vi "GetSensorGroupEndpoints.vi"(11 "SensorGroupId":string) -> (3 "Endpoints out":T1[](array[typedef]))   [LabVIEW 2017, in "DeviceModelHelpers.lvlib"]
uses:
  <vilib>/addons/InsightCM/Utilities/DeviceModelHelpers/DeviceModelHelpers.lvlib
  <vilib>/addons/InsightCM/MessageBus/Base/controls/WirelessEndpoint.ctl
  <vilib>/addons/InsightCM/MessageBus/Base/controls/KeyValuePair.ctl
  <vilib>/addons/InsightCM/MessageBus/Base/controls/WirelessChannel.ctl
  <vilib>/addons/InsightCM/Utilities/GlobalConfiguration/GlobalConfiguration.lvlib
  <vilib>/addons/InsightCM/Utilities/PropertyHelpers/PropertyHelpers.lvlib
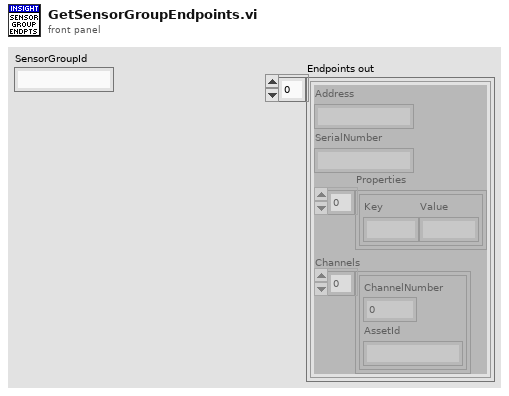
[diagram p1: front panel]
types:
  T1 = typedef "WirelessEndpoint.ctl" = cluster{"Address":string, "SerialNumber":string, "Properties":T2[], "Channels":T3[]}
  T2 = typedef "KeyValuePair.ctl" = cluster{"Key":string, "Value":string}
  T3 = typedef "WirelessChannel.ctl" = cluster{"ChannelNumber":i32, "AssetId":string}
  T4 = typedef "R2_Device.ctl" = cluster{"Id":string, "Name":string, "DeviceType":string, "HardwareName":string, "IpAddress":string, "HardwareInfo":T2[], "ApplicationType":string, "ApplicationVersion":string, "EquipmentIds":string[], "ConfigurationVersion":string, "State":T5, "Properties":T2[], "DataGroups":T6[], "BurstModeTrigger":T10, "SensorGroups":T11[], "Endpoints":T1[]}
  T5 = typedef "DeviceState.ctl" = cluster{"Disabled":bool}
  T6 = typedef "R2_DataGroup.ctl" = cluster{"Name":string, "OperatingStates":T7[], "Properties":T2[], "EquipmentIds":string[], "AssetNodeId":string}
  T7 = typedef "OperatingState.ctl" = cluster{"Name":string, "Properties":T2[], "Triggers":T8[]}
  T8 = typedef "Trigger.ctl" = cluster{"Type":string, "Expression":string, "Conditions":T9[]}
  T9 = typedef "Condition.ctl" = cluster{"Source":string, "Type":string, "Operator":string, "CompareTo":string, "DwellSeconds":dbl}
  T10 = typedef "BurstModeTrigger.ctl" = cluster{"Trigger":T8, "SampleRate":string, "AcquisitionLength":string}
  T11 = typedef "DeviceSensorGroup.ctl" = cluster{"EquipId":string, "SensorGroupId":string}
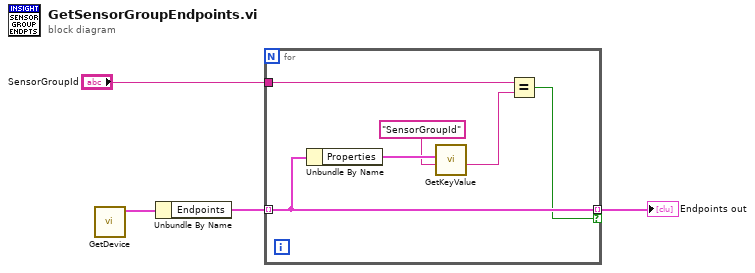
[diagram p0: block diagram]
diagram:
  n1 = call <vilib>:"GetDevice.vi"() -> ("device configuration"=w4:T4)  [unwired: 9 in, 2 out]
  n2 = Unbundle By Name(w4) -> ("Endpoints"=w3:T1[])
  n3 = for {
    tunnel: w3 -> [w6] mode=indexing
    tunnel: "SensorGroupId" -> [w8]
    tunnel: [w6] -> w1 mode=indexing if=w5
    n4 = Unbundle By Name(w6) -> ("Properties"=w10:T2[])
    n5 = call <vilib>:"GetKeyValue.vi"("key"="SensorGroupId", "key value pairs"=w10) -> ("value"=w7:string)  [unwired: 7 in, 2 out]
    n6 = Equal?(x=w8, y=w7) -> (x = y?=w5:bool)
  }
  "Endpoints out" <- w1
